vi "Post Build Script (manual build).vi"(8 "Package Source Folder":path=path "C:/user/patrick/git/Multichannel-Lockin/src", 9 "Package Version":string="2.8.9.18", 10 "Product Name":string="Multichannel Lockin", 11 "Output Package File Path":path) -> (0 "error out":errorcluster)   [LabVIEW 2016, in "PostBuildSupport (2013).lvclass"]
uses:
  PostBuildSupport (2013).lvclass
  PostBuildSupport (2013).lvclass/PostBuildSupport (2013).ctl
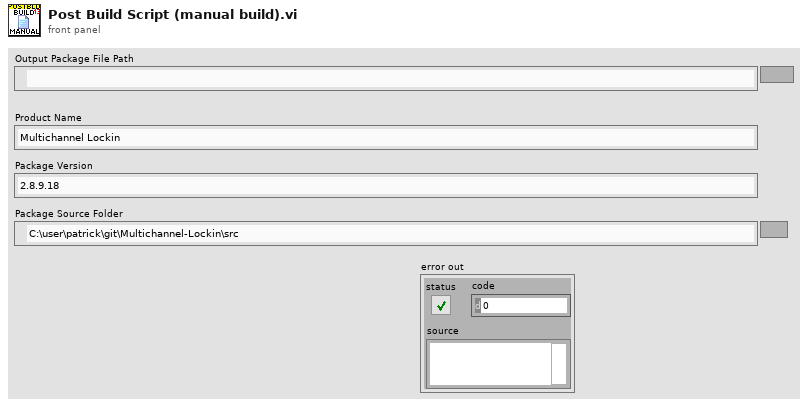
[diagram p1: front panel]
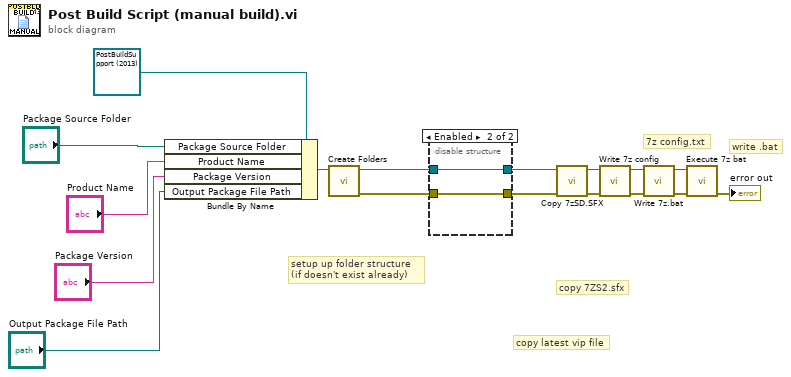
[diagram p0: block diagram]
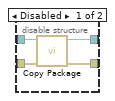
[diagram p2: hidden frame]
diagram:
  # "copy 7ZS2.sfx"
  # "setup up folder structure \n(if doesn't exist already)"
  # "copy latest vip file"
  # "7z config.txt"
  # "write .bat"
  n1 = Bundle By Name(cluster=refnum<class "PostBuildSupport (2013).lvclass"> refnum ("PostBuildSupport in"), "Package Source Folder"="Package Source Folder", "Product Name"="Product Name", "Package Version"="Package Version", "Output Package File Path"="Output Package File Path") -> (w1:refnum<class "PostBuildSupport (2013).lvclass">)
  n2 = call "Create Folders.vi"("PostBuildSupport in"=w1) -> ("error out"=w3:errorcluster, "PostBuildSupport out"=w10:refnum<class "PostBuildSupport (2013).lvclass">)  [unwired: 9 in]
  n3 = disable-structure shown="Enabled" {
    disable-tunnel: w10 -> [w21 w23]
    disable-tunnel: [w20 w23] -> w9
    disable-tunnel: w3 -> [w19 w22]
    disable-tunnel: [w18 w22] -> w2
    frame Disabled {
      n4 = call "Copy Package.vi"("error in (no error)"=w19, "PostBuildSupport in"=w21) -> ("error out"=w18:errorcluster, "PostBuildSupport out"=w20:refnum<class "PostBuildSupport (2013).lvclass">)  [unwired: 8 in]
    }
    frame Enabled {
    }
  }
  n5 = call "Copy 7zSD.SFX.vi"("error in (no error)"=w2, "PostBuildSupport in"=w9) -> ("error out"=w6:errorcluster, "PostBuildSupport out"=w5:refnum<class "PostBuildSupport (2013).lvclass">)  [unwired: 8 in]
  n6 = call "Write 7z config.vi"("error in (no error)"=w6, "PostBuildSupport in"=w5) -> ("error out"=w16:errorcluster, "PostBuildSupport out"=w17:refnum<class "PostBuildSupport (2013).lvclass">)  [unwired: 8 in]
  n7 = call "Write 7z.bat.vi"("error in (no error)"=w16, "PostBuildSupport in"=w17) -> ("error out"=w7:errorcluster, "PostBuildSupport out"=w4:refnum<class "PostBuildSupport (2013).lvclass">)  [unwired: 8 in]
  n8 = call "Execute 7z bat.vi"("error in (no error)"=w7, "PostBuildSupport in"=w4) -> ("error out"=→"error out":errorcluster)  [unwired: 8 in, 1 out]
